vi "Base Sender.vi"() -> (2 "Sender":refnum<class "Sender.lvclass">)   [LabVIEW 2020, in "jettl.lvlib" / "Sender.lvlib"]
uses:
  Sender.lvlib
  Sender/Sender.lvclass
  Base Sender/Base Sender.lvclass
  C:/git/jettl/src/jettl/jettl/Sender/Sender/Sender.lvclass
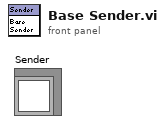
[diagram p1: front panel]
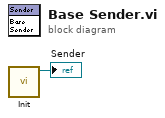
[diagram p0: block diagram]
diagram:
  n1 = call "Init.vi"() -> ("Base Sender out"=→"Sender":refnum<class "Base Sender.lvclass">)  [unwired: 11 in]
